vi "N5765A_STTOPowerOn.vi"(8 "error in (no error)":errorcluster, 10 "STTO Current Limit (amps)":dbl format="%^.3e", 11 "VISA resource name":refnum<visa-resource-name>) -> (0 "error out":errorcluster, 2 "True = STTO":bool, 3 "VISA resource name out":refnum<visa-resource-name>)   [LabVIEW 2015]
doc: "This will program the power supply to 5 volts, and curernt limit to STTO Current Limit and verifies the Power supply is not current limiting"
panel:
  out "Output Voltage":dbl format="%.4f"
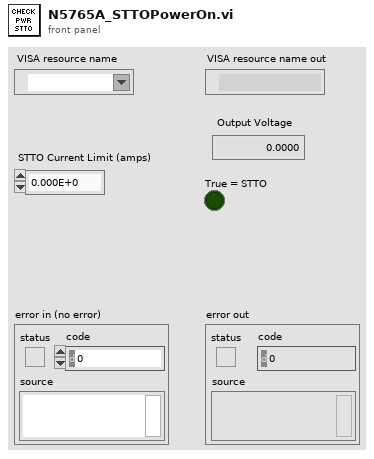
[diagram p1: front panel]
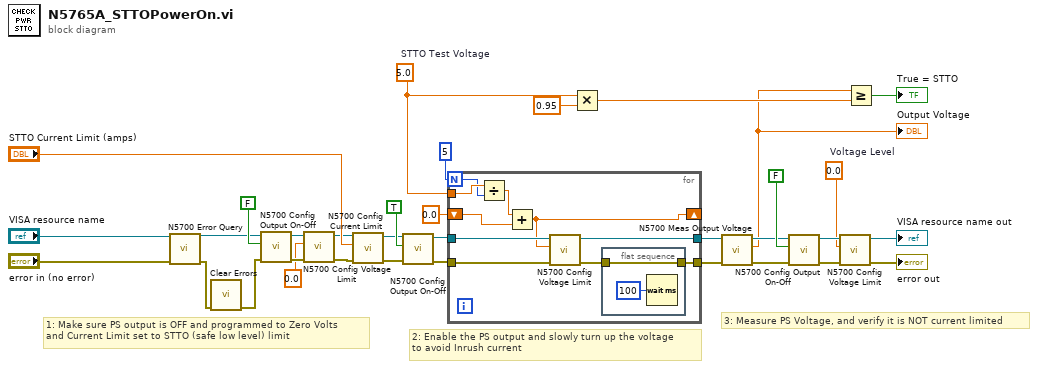
[diagram p0: block diagram]
diagram:
  w17 = 0.0  # Voltage Level
  w11 = 5.0  # STTO Test Voltage
  # "3: Measure PS Voltage, and verify it is NOT current limited"
  # "2: Enable the PS output and slowly turn up the voltage \nto avoid Inrush current"
  # "1: Make sure PS output is OFF and programmed to Zero Volts\nand Current Limit set to STTO (safe low level) limit"
  n1 = call <instrlib>:"N5700 Error Query.vi"("VISA"="VISA resource name", "error"="error in (no error)") -> ("VISA out"=w27:refnum<visa-resource-name>, "error out"=w34:errorcluster)  [unwired: 10 in, 2 out]
  n2 = call <vilib>:"Clear Errors.vi"("error in (no error)"=w34) -> ("error out"=w26:errorcluster)  [unwired: 5 in, 1 out]
  n3 = call <instrlib>:"N5700 Config Output On-Off.vi"("error"=w26, "Output ON"=FALSE ("Enable Output (False)"), "VISA"=w27) -> ("error out"=w8:errorcluster, "VISA out"=w9:refnum<visa-resource-name>)  [unwired: 4 in]
  n4 = call <instrlib>:"N5700 Config Voltage Limit.vi"("error"=w8, "Volt Limit"=0.0, "VISA"=w9) -> ("error out"=w5:errorcluster, "VISA out"=w6:refnum<visa-resource-name>)  [unwired: 4 in]
  n5 = call <instrlib>:"N5700 Config Current Limit.vi"("error"=w5, "Current Limit"="STTO Current Limit (amps)", "VISA"=w6) -> ("error out"=w31:errorcluster, "VISA out"=w32:refnum<visa-resource-name>)  [unwired: 4 in]
  n6 = call <instrlib>:"N5700 Config Output On-Off.vi"("error"=w31, "Output ON"=TRUE ("Enable Output (False)"), "VISA"=w32) -> ("error out"=w3:errorcluster, "VISA out"=w4:refnum<visa-resource-name>)  [unwired: 4 in]
  n7 = for {
    N: 5 -> [w40]
    tunnel: w4 -> [w43]
    tunnel: [w44] -> w2
    tunnel: w3 -> [w42]
    tunnel: [w35] -> w1
    tunnel: w11 -> [w41]
    shift-right: [w37] -> _
    shift-left: 0.0 -> [w38]
    n8 = Divide(x=w41, y=w40) -> (x/y=w39:dbl)
    n9 = Add(x=w39, y=w38) -> (x+y=w37:dbl)
    n10 = call <instrlib>:"N5700 Config Voltage Limit.vi"("error"=w42, "Volt Limit"=w37, "VISA"=w43) -> ("error out"=w36:errorcluster, "VISA out"=w44:refnum<visa-resource-name>)  [unwired: 4 in]
    n11 = flat-sequence {
      tunnel: w36 -> [w45]
      tunnel: [w45] -> w35
      frame #0 {
        n12 = Wait (ms)(milliseconds to wait=u32 100) -> ()  [unwired: 1 out]
      }
    }
  }
  n13 = Multiply(x=w11, y=0.95) -> (x*y=w14:dbl)
  n14 = call <instrlib>:"N5700 Meas Output Voltage.vi"("error"=w1, "VISA"=w2) -> ("error out"=w20:errorcluster, "Output Voltage"=w13:dbl, "VISA out"=w21:refnum<visa-resource-name>)  [unwired: 4 in]
  "Output Voltage" <- w13
  n15 = call <instrlib>:"N5700 Config Output On-Off.vi"("error"=w20, "Output ON"=FALSE ("Enable Output (False)"), "VISA"=w21) -> ("error out"=w19:errorcluster, "VISA out"=w18:refnum<visa-resource-name>)  [unwired: 4 in]
  n16 = call <instrlib>:"N5700 Config Voltage Limit.vi"("error"=w19, "Volt Limit"=w17, "VISA"=w18) -> ("error out"=→"error out":errorcluster, "VISA out"=→"VISA resource name out":refnum<visa-resource-name>)  [unwired: 4 in]
  n17 = Greater Or Equal?(x=w13, y=w14) -> (x >= y?=→"True = STTO":bool)
